vi "setAxisScaleEngine.vi"(8 "Error In":errorcluster, 9 "engine":refnum<class "QwtScaleEngine.lvclass">, 10 "axisId":T1 items=["YLeft", "YRight", "XBottom", "XTop"], 11 "QwtPlot In":refnum<class "QwtPlot.lvclass">) -> (0 "Error Out":errorcluster, 3 "QwtPlot Out":refnum<class "QwtPlot.lvclass">)   [LabVIEW 2014, in "QwtPlot.lvclass"]
doc: "LabVIEW-specific documentation is not yet available. See <b>https://qwt.sourceforge.io/class_qwt_plot.html#setAxisScaleEngine</b>"
uses:
  QwtPlot.lvclass
  QwtAxis/Position.ctl
  QwtScaleEngine/QwtScaleEngine.lvclass
  LQ Core/LQIdentity/LQIdentity.lvclass/LQIdentity.ctl
  LQ Core/LQ Core.lvlib
  LQ Core/LQIdentity/LQIdentity.lvclass
  QwtAxis/QwtAxis.lvlib
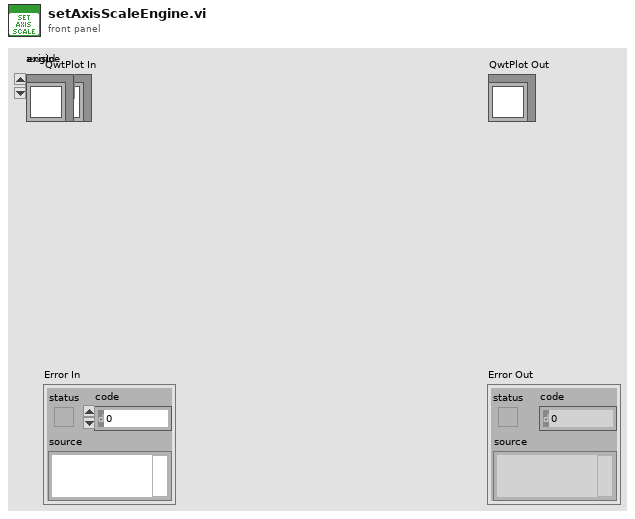
[diagram p1: front panel]
types:
  T1 = typedef "QwtAxis.lvlib/Position.ctl" = i32
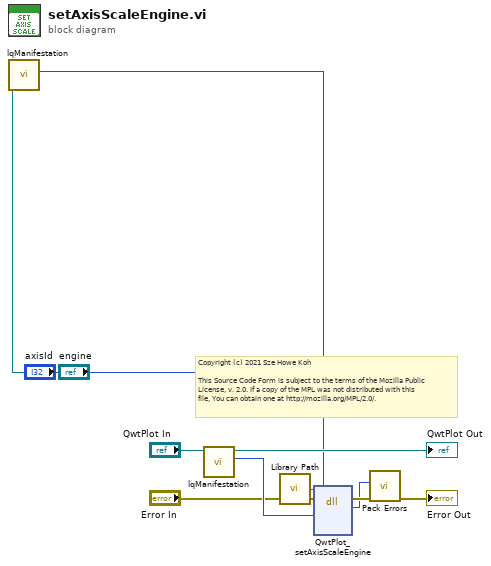
[diagram p0: block diagram]
diagram:
  # "Copyright (c) 2021 Sze Howe Koh\n\nThis Source Code Form is subject to the terms of the Mozilla Public\nLicense, v. 2.0. If a copy of the MPL was not distributed with this\nfile, You can obtain one at http://mozilla.org/MPL/2.0/."
  n1 = call "lqManifestation.vi"("LQIdentity in"="engine") -> ("Manifestation"=w1:u64)  [unwired: 9 in, 1 out]
  n2 = call "lqManifestation.vi"("LQIdentity in"="QwtPlot In") -> ("Manifestation"=w8:u64, "LQIdentity out"=→"QwtPlot Out":refnum<class "QwtPlot.lvclass">)  [unwired: 9 in]
  n3 = call "Library Path.vi"() -> ("Library Path"=w9:path)
  n4 = dll-call lib="?" fn="QwtPlot_setAxisScaleEngine"(path in=w9, error in="Error In", "_instance"=w8, "axisId"="axisId", "engine"=w1) -> (error out=w6:errorcluster, w4:i32)  [unwired: 4 in, 1 out]
  n5 = call "Pack Errors.vi"("Error In"=w6, "Error Code"=w4) -> ("Error Out"=→"Error Out":errorcluster)  [unwired: 9 in]
